vi "TAFTraceWindow_ClassCast.vi"(11 "TAFTraceWindow in":refnum<class>) -> (3 "TAFTraceWindow out":refnum<class "TAFTraceWindow.lvclass">)   [LabVIEW 2021, in "TAFTraceWindow.lvclass"]
uses:
  TAFTraceWindow.lvclass
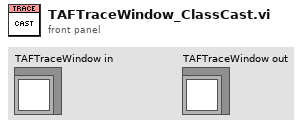
[diagram p1: front panel]
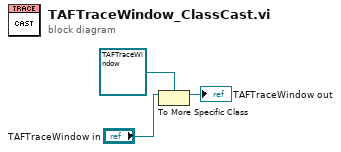
[diagram p0: block diagram]
diagram:
  n1 = To More Specific Class(target class=refnum<class "TAFTraceWindow.lvclass"> refnum ("reference in"), reference="TAFTraceWindow in") -> (specific class reference=→"TAFTraceWindow out":refnum<class "TAFTraceWindow.lvclass">)  [unwired: 1 in, 1 out]
